vi "Release Queue.vi"(8 "error in (no error)":errorcluster) -> (0 "error out":errorcluster)   [LabVIEW 2023, in "Template.lvlib"]
doc: "VI used to release the queue used in the module."
uses:
  Template.lvlib
  Type Def/FGV Queue State.ctl
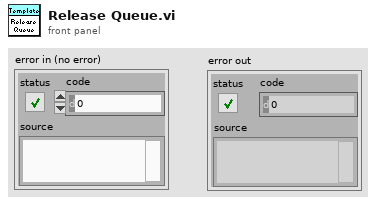
[diagram p1: front panel]
types:
  T1 = typedef "Template.lvlib/FGV Queue State.ctl" = enum16{"Get", "Set"}
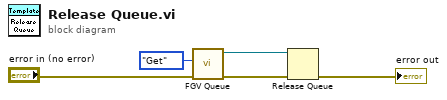
[diagram p0: block diagram]
diagram:
  n1 = call "FGV Queue.vi"("error in (no error)"="error in (no error)", "FGV Queue State"=FGV_Queue_State."Get") -> ("error out"=w2:errorcluster, "queue out"=w3:refnum<queue>)  [unwired: 8 in]
  n2 = Release Queue(queue=w3, error in (no error)=w2) -> (error out=→"error out":errorcluster)  [unwired: 1 in, 2 out]
